vi "Run ACS.vi"(8 "error in (no error)":errorcluster, 11 "AutoExp in":refnum<class "AutoExp.lvclass">) -> (0 "error out":errorcluster, 3 "AutoExp out":refnum<class "AutoExp.lvclass">)   [LabVIEW 2018, in "AutoExp.lvclass"]
uses:
  AutoExp.lvclass
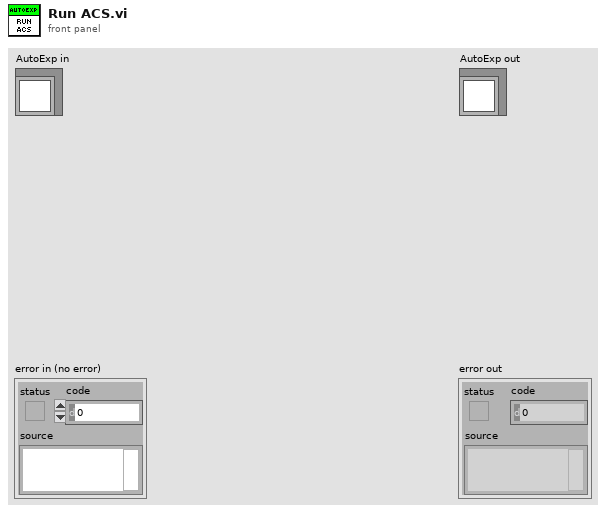
[diagram p1: front panel]
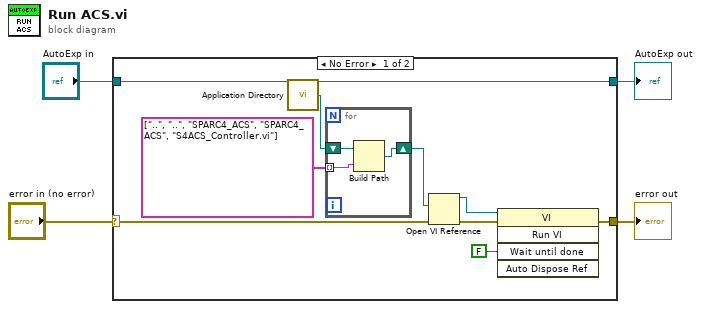
[diagram p0: block diagram]
diagram:
  n1 = case shown="No Error" "error in (no error)" {
    selector: "error in (no error)" -> [w8 w18]
    tunnel: [w6 w18] -> w3
    tunnel: [w13 w17] -> w1
    tunnel: "AutoExp in" -> [w13 w17]
    frame No Error {
      n2 = call <vilib>:"Application Directory.vi"() -> ("Application Directory"=w5:path)
      n3 = for {
        tunnel: string[] ["..", "..", "SPARC4_ACS", "SPARC4_ACS", "S4ACS_Controller.vi"] -> [w14] mode=indexing
        shift-right: [w16] -> w7
        shift-left: w5 -> [w15]
        n4 = Build Path(base path=w15, name or relative path=w14) -> (appended path=w16:path)
      }
      n5 = Open VI Reference(vi path=w7, error in (no error)=w8) -> (vi reference=w11:refnum<vi>, error out=w10:errorcluster)  [unwired: 4 in]
      n6 = invoke class="VI" method="Run VI"(reference=w11, error in=w10, "Wait until done"=FALSE ("Wait Until Done")) -> (error out=w6:errorcluster)  [unwired: 2 in, 4 out]
    }
    frame Error {
    }
  }
  "error out" <- w3
  "AutoExp out" <- w1
